vi "ArrayColorU64ToImage.vi"(8 "error in":errorcluster, 10 "Pixel":u64[][](array[numeric]), 11 "Image Reference In":T1) -> (0 "error out":errorcluster, 3 "Image Reference Out":T1)   [LabVIEW 2024, in "OpenLvVision_Image.lvlib" / "DataAccess.lvlib"]
doc: "Replaces the image's data with the provided array (Copy)"
uses:
  DataAccess.lvlib
  Management/TypeDef/Image.ctl
  TypeDef/StepSizes.ctl
  Management/Management.lvlib
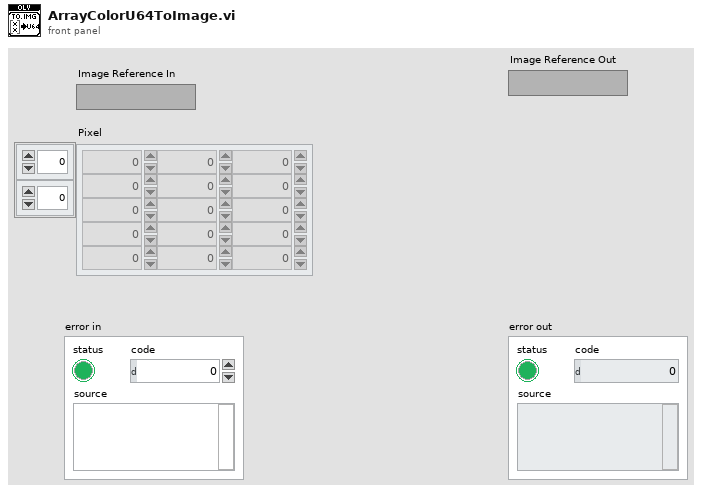
[diagram p1: front panel]
types:
  T1 = typedef "OpenLvVision_Image.lvlib/Management.lvlib/Image.ctl" = refnum<image>
  T2 = typedef "OpenLvVision_Image.lvlib/DataAccess.lvlib/StepSizes.ctl" = cluster{"X Step Size":u32, "Y Step Size":u32}
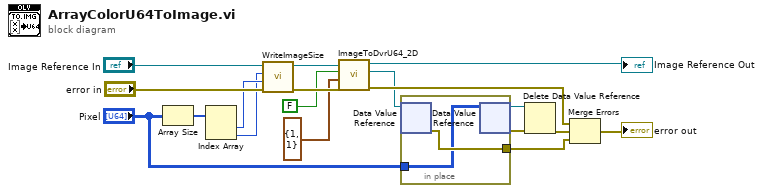
[diagram p0: block diagram]
diagram:
  n1 = Array Size(array="Pixel") -> (size(s)=w4:i32[])
  n2 = Index Array(array=w4) -> (element #1=w3:i32, element #2=w2:i32)  [unwired: 2 in]
  n3 = call "WriteImageSize.vi"("error in"="error in", "Height"=w3, "Width"=w2, "Image Reference In"="Image Reference In") -> ("error out"=w15:errorcluster, "Image Reference Out"=w16:T1)  [unwired: 6 in]
  n4 = call "ImageToDvrU64_2D.vi"("error in"=w15, "Step Sizes"=T2 {"X Step Size"=1, "Y Step Size"=1}, "Include Border"=FALSE, "Image Reference In"=w16) -> ("error out"=w8:errorcluster, "EDVR 2D U64"=w7:refnum<data-value>, "Image Reference Out"=→"Image Reference Out":T1)  [unwired: 4 in, 1 out]
  n5 = in-place {
    in-place-border: [w20] -> w9
    in-place-border: "Pixel" -> [w19]
    n6 = in-place-dvr #1(w7) -> (w20:errorcluster)  [unwired: 1 out]
    n7 = in-place-dvr #1(w19) -> (w13:refnum<data-value>, w12:errorcluster)
  }
  n8 = Delete Data Value Reference(data value reference=w13, error in=w12) -> (error out=w11:errorcluster)  [unwired: 1 out]
  n9 = Merge Errors(w8, w11, w9) -> (→"error out":errorcluster)
